vi "util-address-range.vi"(10 "ADDR":T1 format="%04d") -> (2 "x .and. y?":bool)   [LabVIEW 2024]
uses:
  controls/type.address.ctl
panel:
  out "Port Number":u8 format="%02d"
  out "Device Address":u8 format="%02d"
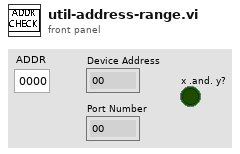
[diagram p1: front panel]
types:
  T1 = typedef "type.address.ctl" = u16
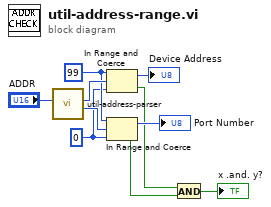
[diagram p0: block diagram]
diagram:
  w7 = u8 99 ("lower limit")
  w6 = u8 0 ("lower limit")
  n1 = call "util-address-parser.vi"("ADDR 2"="ADDR") -> ("Channel"=w8:u8, "Address"=w9:u8)  [unwired: 9 in]
  n2 = In Range and Coerce(upper limit=w7, x=w9, lower limit=w6) -> (coerced(x)=→"Device Address":u8, In Range?=w3:bool)
  n3 = In Range and Coerce(upper limit=w7, x=w8, lower limit=w6) -> (coerced(x)=→"Port Number":u8, In Range?=w2:bool)
  n4 = And(x=w3, y=w2) -> (x .and. y?=→"x .and. y?":bool)
